vi "globalSetUp.vi"(8 "error in":errorcluster, 11 "Loopback in":refnum<class "Loopback.lvclass">) -> (0 "error out":errorcluster, 3 "Loopback out":refnum<class "Loopback.lvclass">)   [LabVIEW 2020, in "Loopback.lvclass"]
uses:
  Loopback.lvclass
  Shared/Device Parameters.ctl
  Shared/Initialization Method.ctl
  Shared/Bus Selection.ctl
  Shared/Coupling Mode.ctl
  Loopback.lvclass/Loopback.ctl
  niveristand-custom-device-testing-tools/VeriStandTestUtilities/VeriStandTestUtilities.lvlib
  Scripting/AIM MIL-STD-1553 Scripting.lvlib
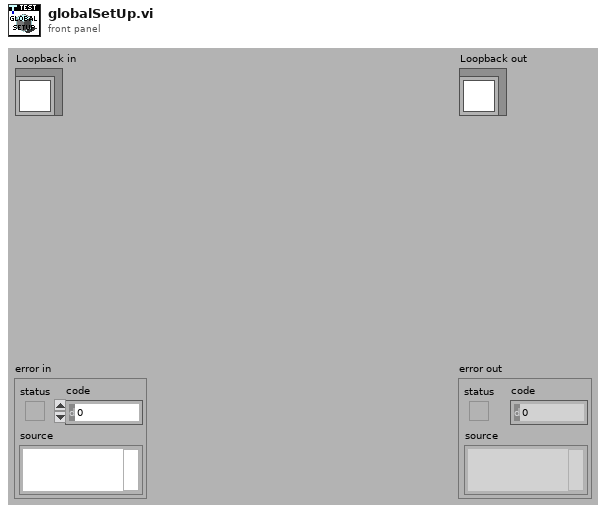
[diagram p1: front panel]
types:
  T1 = typedef "Device Parameters.ctl" = cluster{"initialization method":T2, "card number":i32, "pxi slot number":i32, "biu number":i32, "bus selection":T3, "coupling mode":T4}
  T2 = typedef "Initialization Method.ctl" = enum16{"PXI Slot Number", "Card Number"}
  T3 = typedef "Bus Selection.ctl" = enum16{"Both", "Primary", "Secondary"}
  T4 = typedef "Coupling Mode.ctl" = enum16{"Isolated Onboard Termination", "Transformer Coupled", "Direct Coupled", "External with Onboard Termination", "Onboard Digital Wrap-around"}
  T5 = typedef "Custom Device API.lvlib/Custom Device Item Ref.ctl" = u64
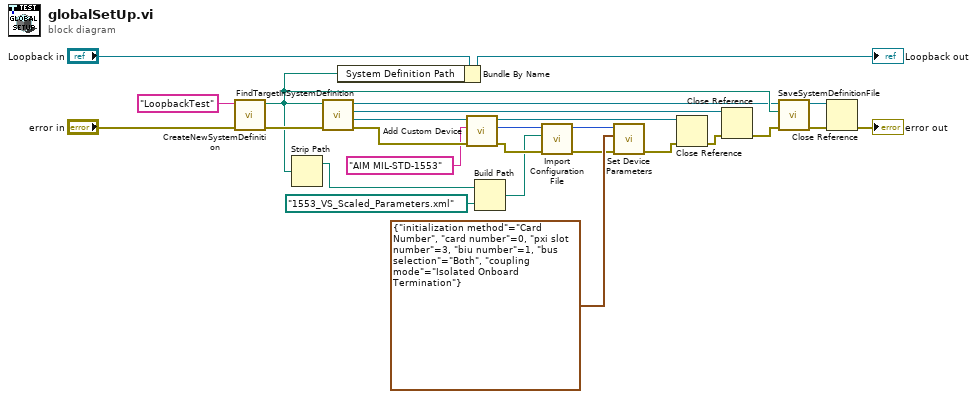
[diagram p0: block diagram]
diagram:
  n1 = call "CreateNewSystemDefinition.vi"("error in"="error in", "System Definition Name"="LoopbackTest") -> ("error out"=w26:errorcluster, "System Definition Path"=w25:path)  [unwired: 8 in]
  n2 = Strip Path(path=w25) -> (stripped path=w6:path)  [unwired: 1 out]
  n3 = call "FindTargetInSystemDefinition.vi"("error in"=w26, "system definition path"=w25) -> ("error out"=w21:errorcluster, "Target"=w15:refnum<k24>, "Root"=w16:refnum<k24>, "System Definition"=w14:refnum<k24>)  [unwired: 6 in]
  n4 = Bundle By Name(cluster="Loopback in", "System Definition Path"=w25) -> (→"Loopback out":refnum<class "Loopback.lvclass">)
  n5 = call "Add Custom Device.vi"("error in"=w21, "custom device name"="AIM MIL-STD-1553" ("name"), "target"=w15) -> ("error out"=w9:errorcluster, "custom device ref out"=w8:T5, "target out"=w18:refnum<k24>)  [unwired: 6 in]
  n6 = Build Path(base path=w6, name or relative path=path "1553_VS_Scaled_Parameters.xml") -> (appended path=w5:path)
  n7 = call "Import Configuration File.vi"("error in"=w9, "parameters configuration file path"=w5, "custom device ref"=w8) -> ("error out"=w3:errorcluster, "custom device ref out"=w1:T5)  [unwired: 7 in]
  n8 = call "Set Device Parameters.vi"("error in"=w3, "device parameters"=T1 {"initialization method"=enum."Card Number", "card number"=0, "pxi slot number"=3, "biu number"=1, "bus selection"=enum."Both", "coupling mode"=enum."Isolated Onboard Termination"}, "custom device"=w1) -> ("error out"=w2:errorcluster)  [unwired: 7 in, 1 out]
  n9 = Close Reference(reference=w18, error in (no error)=w2) -> (error out=w19:errorcluster)
  n10 = Close Reference(reference=w16, error in (no error)=w19) -> (error out=w17:errorcluster)
  n11 = call "SaveSystemDefinitionFile.vi"("error in (no error)"=w17, "System Definition File in"=w25, "System Definition Reference in"=w14) -> ("error out"=w22:errorcluster, "System Definition Reference out"=w23:refnum<k24>)  [unwired: 7 in]
  n12 = Close Reference(reference=w23, error in (no error)=w22) -> (error out=→"error out":errorcluster)
